vi "ParseMotorData.vi"(8 "error in (no error)":errorcluster, 9 "TPDO data":u8[](array[numeric]), 10 "PDO channel":u8(ring) items=["PDO 1", "PDO 2", "PDO 3", "PDO 4"], 11 "MotorController in":refnum<class "MotorController.lvclass">) -> (0 "error out":errorcluster, 3 "MotorController out":refnum<class "MotorController.lvclass">)   [LabVIEW 2017, in "MotorController.lvclass"]
uses:
  MotorController.lvclass
  MotorController.lvclass/MotorController.ctl
  <vilib>/CANopenLib/CANOPEN.llb/CANopen Fetch from Data [U16].vi
  <vilib>/CANopenLib/CANOPEN.llb/CANopen Fetch from Data [I32].vi
  <vilib>/CANopenLib/CANOPEN.llb/CANopen Fetch from Data [U8].vi
  <vilib>/CANopenLib/CANOPEN.llb/CANopen Fetch from Data [I16].vi
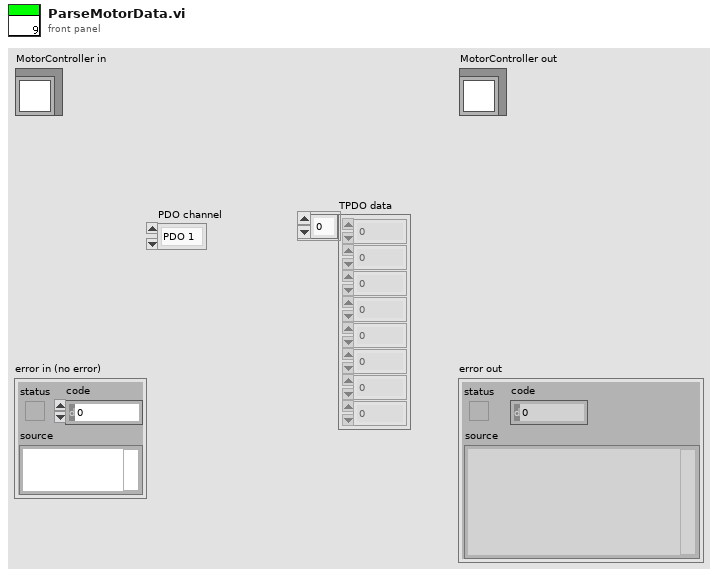
[diagram p1: front panel]
types:
  T1 = typedef "MotorData.ctl" = cluster{"Velo (RPM)":i32, "MotorTemp(C)":u8, "CtrlTemp(C)":u8, "DcLinkVolt(V)":dbl, "ErrorCode":dbl, "isAlive":bool, "motorControllerState":u16, "motorStatus":T2}
  T2 = typedef "MotorStatus.ctl" = cluster{"isReady":bool, "isOn":bool, "isOperEn":bool, "isFault":bool, "isVoltEn":bool, "targetReached":bool, "isWarning":bool}
  T3 = cluster{"isReady":bool, "isOn":bool, "isOperEn":bool, "isFault":bool, "isVoltEn":bool, "targetReached":bool, "isWarning":bool}
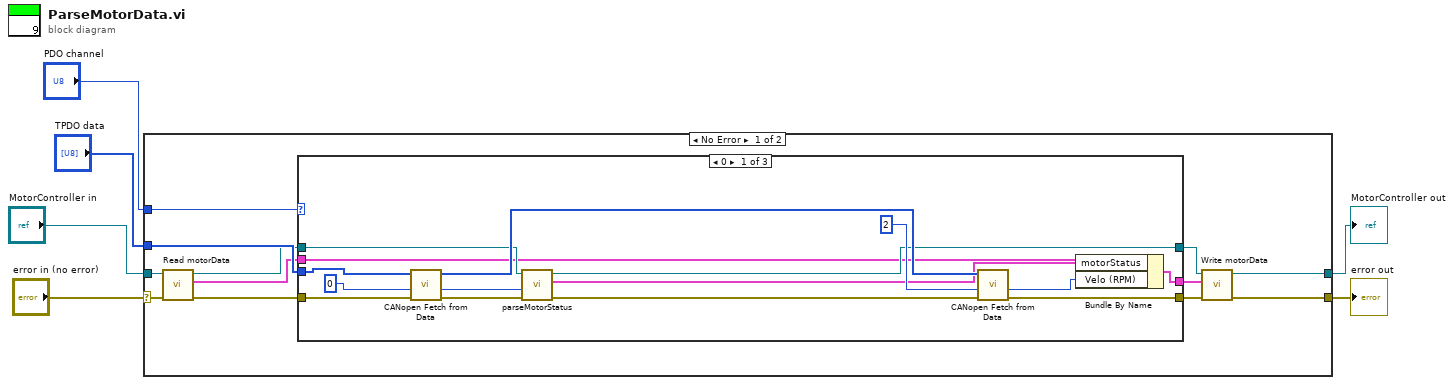
[diagram p0: block diagram]
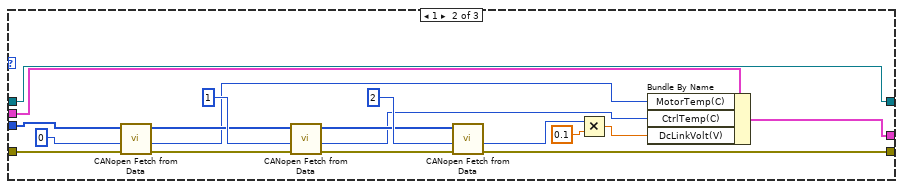
[diagram p2: hidden frame]
diagram:
  n1 = case shown="No Error" "error in (no error)" {
    selector: "error in (no error)" -> [w17 w56]
    tunnel: [w11 w56] -> w5
    tunnel: [w10 w55] -> w3
    tunnel: "MotorController in" -> [w15 w55]
    tunnel: "PDO channel" -> [w18 _]
    tunnel: "TPDO data" -> [w16 _]
    frame No Error {
      n2 = call "Read motorData.vi"("error in (no error)"=w17, "MotorController in"=w15) -> ("error out"=w9:errorcluster, "motorData"=w14:T1, "MotorController out"=w8:refnum<class "MotorController.lvclass">)  [unwired: 7 in]
      n3 = case shown="0" w18 {
        tunnel: w16 -> [w32 w47 _]
        tunnel: w9 -> [w22 w45 w53]
        tunnel: w14 -> [w23 w44 w54]
        tunnel: [w21 w39 w53] -> w13
        tunnel: [w25 w43 w54] -> w12
        tunnel: w8 -> [w24 w42 w52]
        tunnel: [w26 w42 w52] -> w7
        frame 0 {
          n4 = call-poly <vilib>:"CANopen Fetch from Data.vi"("error in (no error)"=w22, "offset (0)"=u32 0, "CANopen data in"=w32) -> ("error out"=w28:errorcluster, "unsigned 16-bit integer"=w29:u16, "CANopen data out"=w31:u8[])  [unwired: 6 in]
          n5 = call "parseMotorStatus.vi"("error in (no error)"=w28, "inputStatus"=w29, "MotorController in"=w24) -> ("error out"=w27:errorcluster, "output cluster"=w19:T3, "MotorController out"=w26:refnum<class "MotorController.lvclass">)  [unwired: 6 in]
          n6 = call-poly <vilib>:"CANopen Fetch from Data.vi"("error in (no error)"=w27, "offset (0)"=u32 2, "CANopen data in"=w31) -> ("error out"=w21:errorcluster, "signed 32-bit integer"=w20:i32)  [unwired: 6 in, 1 out]
          n7 = Bundle By Name(cluster=w23, "motorStatus"=w19, "Velo (RPM)"=w20) -> (w25:T1)
        }
        frame 1 {
          n8 = call-poly <vilib>:"CANopen Fetch from Data.vi"("error in (no error)"=w45, "offset (0)"=u32 0, "CANopen data in"=w47) -> ("error out"=w49:errorcluster, "unsigned 8-bit integer"=w35:u8, "CANopen data out"=w48:u8[])  [unwired: 6 in]
          n9 = call-poly <vilib>:"CANopen Fetch from Data.vi"("error in (no error)"=w49, "offset (0)"=u32 1, "CANopen data in"=w48) -> ("error out"=w40:errorcluster, "unsigned 8-bit integer"=w34:u8, "CANopen data out"=w36:u8[])  [unwired: 6 in]
          n10 = call-poly <vilib>:"CANopen Fetch from Data.vi"("error in (no error)"=w40, "offset (0)"=u32 2, "CANopen data in"=w36) -> ("error out"=w39:errorcluster, "signed 16-bit integer"=w37:i16)  [unwired: 6 in, 1 out]
          n11 = Multiply(x=w37, y=0.1) -> (x*y=w38:dbl)
          n12 = Bundle By Name(cluster=w44, "MotorTemp(C)"=w35, "CtrlTemp(C)"=w34, "DcLinkVolt(V)"=w38) -> (w43:T1)
        }
        frame Default {
        }
      }
      n13 = call "Write motorData.vi"("error in (no error)"=w13, "motorData"=w12, "MotorController in"=w7) -> ("error out"=w11:errorcluster, "MotorController out"=w10:refnum<class "MotorController.lvclass">)  [unwired: 7 in]
    }
    frame Error {
    }
  }
  "error out" <- w5
  "MotorController out" <- w3
